vi "Tool_Unicode Property Interpret As Unicode.vi"(7 "Interpret As Unicode (T)":bool=TRUE, 8 "error in (no error)":errorcluster, 9 "String Control Reference":refnum<vi>) -> (2 "error out":errorcluster, 3 "String Control Reference":refnum<vi>)   [LabVIEW 2009]
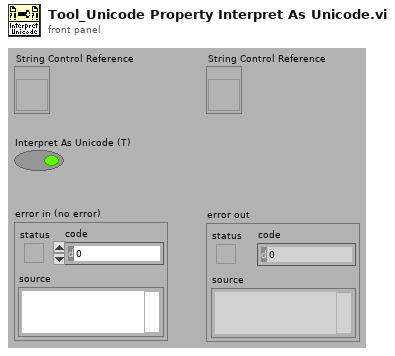
[diagram p1: front panel]
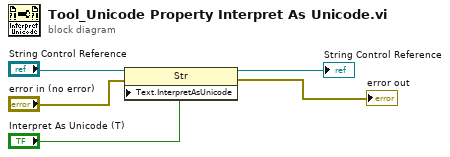
[diagram p0: block diagram]
diagram:
  n1 = property class="Str"(reference="String Control Reference", error in="error in (no error)", "Text.InterpretAsUnicode"="Interpret As Unicode (T)") -> (reference out=→"String Control Reference":refnum<vi>, error out=→"error out":errorcluster)
